vi "gfitsio-read-image-subset-dbl-2d.vi"(4 "npixels (rest)":i32[](array[numeric]), 6 "fpixel (origin)":i32[](array[numeric]), 7 "inc (1)":i32[](array[numeric]), 8 "error in (no error)":errorcluster, 11 "gfits refnum":T1) -> (0 "error out":errorcluster, 2 "data":dbl[][](array[numeric]), 3 "dup gfits refnum":T1)   [LabVIEW 2024, in "gfitsio.lvlib"]
doc: "Read a rectangular subset of the FITS data array. <B>fpixel</B>, <b>npixels</b>, and <b>inc</b> must have the same number of elements as the image has dimensions. <b>fpixel</b> specifies the first pixel in the subset. <b>npixels</b> specifies the number of pixels to read along each image dimension, and should be at least 1 for each dimension. The number of elements greater than 1 in <b>npixels</b> determines the dimensionality of the resulting array, and should match the dimensions of the array returned by the particular instance of the polymorphic GFITSIO read function used. <b>inc</b> specifies the decimation to use along each dimension of the image. 2 will read every other pixel, 3 will read every third pixel, and so on. <B>fpixel</B>, <b>npixels</b>, and <b>inc</b> must be specified in ROW-MAJOR order, with the fastest changing dimension (NAXIS1) listed last and the slowest changing dimension listed first. The array that is returned will be structured according to <B>npixels</B>. For example, a 4 dimensional image is stored in a FITS file and read with <b>npixels</b> = [1, 4, 1, 5]. A two dimensional array will be returned with 5 columns and 4 rows. The column dimension in LabVIEW will correspond to NAXIS1 and the row dimension in LabVIEW will correspond to NAXIS3. <b>fpixel</b> will specify the particular pixel along NAXIS2 and NAXIS4 used for the read and it will specify the starting pixel for NAXIS1 and NAXIS3."
uses:
  gfitsio.lvlib
  gfitsio-refnum.ctl
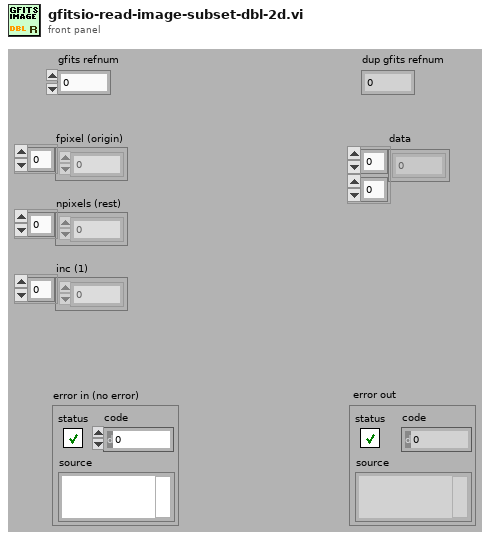
[diagram p1: front panel]
types:
  T1 = typedef "gfitsio.lvlib/gfitsio-refnum.ctl" = u64
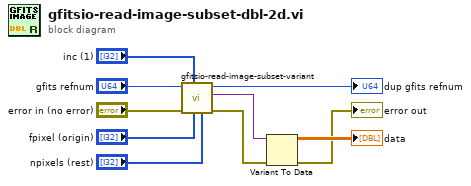
[diagram p0: block diagram]
diagram:
  n1 = call "gfitsio-read-image-subset-variant.vi"("npixels (rest)"="npixels (rest)", "fpixel (origin)"="fpixel (origin)", "inc (1)"="inc (1)", "error in (no error)"="error in (no error)", "gfits refnum"="gfits refnum") -> ("error out"=w5:errorcluster, "Variant"=w7:variant, "dup gfits refnum"=→"dup gfits refnum":T1)  [unwired: 4 in]
  n2 = Variant To Data(error in=w5, Variant=w7) -> (data=→"data":dbl[][], error out=→"error out":errorcluster)  [unwired: 1 in]
